vi "spec_set_ioncounter_state.vi"(8 "error in (no error)":errorcluster, 10 "state (on/off)":bool, 11 "Qtegra in":refnum<class "Qtegra.lvclass">) -> (0 "error out":errorcluster, 2 "return value":string, 3 "Qtegra out":refnum<class "Qtegra.lvclass">)   [LabVIEW 2017, in "Qtegra.lvclass"]
doc: "Activates or deactivates the ion counter\n\nused for qtegra"
uses:
  Qtegra.lvclass
  \\Mac\Home/my data/University/Lamont/Software/LabView/MSControlSuite_Code/MSControl/Classes/Instrument/instrument.lvclass
  global variables.vi
  instrument.lvclass
  StatusLog/StatusLog.lvclass
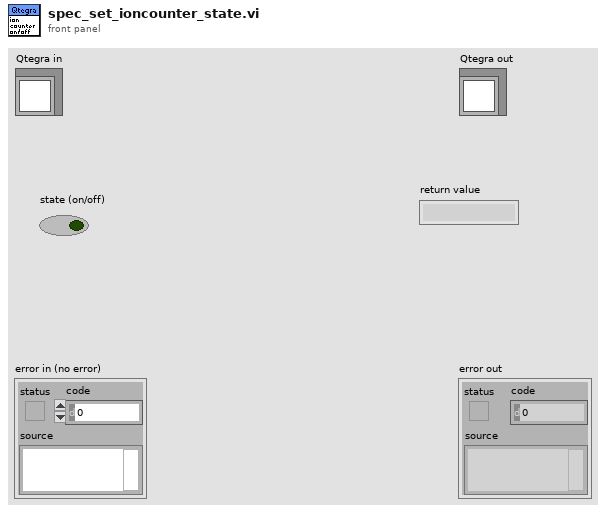
[diagram p1: front panel]
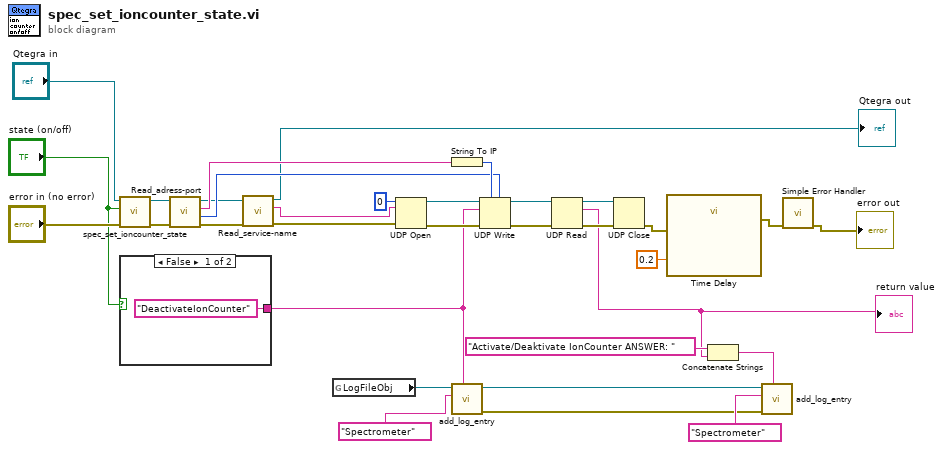
[diagram p0: block diagram]
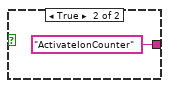
[diagram p2: hidden frame]
diagram:
  n1 = call-parent "spec_set_ioncounter_state.vi"("error in (no error)"="error in (no error)", "state (on/off)"="state (on/off)", "instrument in"="Qtegra in") -> ("error out"=w6:errorcluster, "instrument out"=w7:refnum<class "Qtegra.lvclass">)  [unwired: 6 in, 1 out]
  n2 = case shown="False" "state (on/off)" {
    tunnel: ["DeactivateIonCounter" "ActivateIonCounter"] -> w1
    frame False {
    }
    frame True {
    }
  }
  n3 = call "Read_adress-port.vi"("error in (no error)"=w6, "instrument in"=w7) -> ("error out"=w23:errorcluster, "port number"=w24:i32, "adress"=w31:string, "instrument out"=w22:refnum<class "Qtegra.lvclass">)  [unwired: 6 in]
  n4 = call-dynamic "Read_service-name.vi"("error in (no error)"=w23, "instrument in"=w22) -> ("error out"=w21:errorcluster, "service name"=w20:string, "instrument out"=→"Qtegra out":refnum<class "Qtegra.lvclass">)  [unwired: 7 in]
  n5 = global read "global variables.vi" "LogFileObj"() -> (w12:refnum<class "StatusLog.lvclass">)
  n6 = UDP Open(8:w21, 10:w20, 11:u16 0 ("port")) -> (port=w27:refnum<k16>, 0:w28:errorcluster)  [unwired: 2 in, 1 out]
  n7 = String To IP(1:w31) -> (0:w30:u32)
  n8 = call-dynamic "add_log_entry.vi"("new entry"=w1, "log identifiers"="Spectrometer", "StatusLog in"=w12) -> ("error out"=w8:errorcluster, "StatusLog out"=w11:refnum<class "StatusLog.lvclass">)  [unwired: 5 in]
  n9 = UDP Write(address=w30, port or service name=w24, connection ID=w27, data in=w1, 8:w28) -> (error out=w25:errorcluster, 3:w26:refnum<k16>)  [unwired: 1 in]
  n10 = UDP Read(connection ID=w26, 8:w25) -> (data out=w3:string, error out=w19:errorcluster, 3:w18:refnum<k16>)  [unwired: 2 in, 2 out]
  "return value" <- w3
  n11 = UDP Close(connection ID=w18, 8:w19) -> (error out=w17:errorcluster)  [unwired: 1 out]
  n12 = call "Time Delay"("error in (no error)"=w17, "Delay Time (s)"=0.2) -> ("error out"=w16:errorcluster)  [unwired: 9 in]
  n13 = Concatenate Strings("Activate/Deaktivate IonCounter ANSWER: ", w3) -> (w9:string)
  n14 = call-dynamic "add_log_entry.vi"("new entry"=w9, "error in (no error)"=w8, "log identifiers"="Spectrometer", "StatusLog in"=w11) -> ()  [unwired: 4 in, 2 out]
  n15 = call <vilib>:"Simple Error Handler.vi"("error in (no error)"=w16) -> ("error out"=→"error out":errorcluster)  [unwired: 4 in, 4 out]
